vi "posi incial-proceso 4.vi"() -> ()   [LabVIEW 2020]
panel:
  out "posi incial-proceso 4":T1
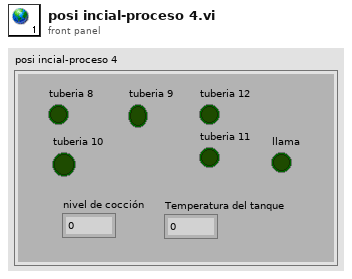
[diagram p1: front panel]
types:
  T1 = cluster{"tuberia 8":bool, "tuberia 9":bool, "tuberia 10":bool, "tuberia 11":bool, "tuberia 12":bool, "nivel de cocción":dbl, "Temperatura del tanque":dbl, "llama":bool}
diagram:
